vi "Build Array String.vi"() -> ()   [LabVIEW 2010]
panel:
  out "new string":string="CP_Data[000]=0x00\\r\nCP_Data[001]=0x00\\r\nCP_Data[002]=0x00\\r\nCP_Data[003]=0x00\\r\nCP_Data[004]=0x00\\r\nCP_Data[005]=0x00\\r\nCP_Data[006]=0x00\\r\nCP_Data[007]=0x00\\r\nCP_Data[008]=0x00\\r\nCP_Data[009]=0x00\\r\nCP_Data[010]=0x00\\r\nCP_Data[011]=0x00\\r\nCP_Data[012]=0x00\\r\nCP_Data[013]=0x00\\r\nCP_Data[014]=0x00\\r\nCP_Data[015]=0x00\\r\nCP_Data[016]=0x00\\r\nCP_Data[017]=0x00\\r\nCP_Data[018]=0x00\\r\nCP_Data[019]=0x00\\r\nCP_Data[020]=0x00\\r\nCP_Data[021]=0x00\\r\nCP_Data[022]=0x00\\r\nCP_Data[023]=0x00\\r\nCP_Data[024]=0x00\\r\nCP_Data[025]=0x00\\r\nCP_Data[026]=0x00\\r\nCP_Data[027]=0x00\\r\nCP_Data[028]=0x00\\r\nCP_Data[029]=0x00\\r\nCP_Data[030]=0x00\\r\nCP_Data[031]=0x00\\r\nCP_Data[032]=0x00\\r\nCP_Data[033]=0x00\\r\nCP_Data[034]=0x00\\r\nCP_Data[035]=0x00\\r\nCP_Data[036]=0x00\\r\nCP_Data[037]=0x00\\r\nCP_Data[038]=0x00\\r\nCP_Data[039]=0x00\\r\nCP_Data[040]=0x00\\r\nCP_Data[041]=0x00\\r\nCP_Data[042]=0x00\\r\nCP_Data[043]=0x00\\r\nCP_Data[044]=0x00\\r\nCP_Data[045]=0x00\\r\nCP_Data[046]=0x00\\r\nCP_Data[047]=0x00\\r\nCP_Data[048]=0x00\\r\nCP_Data[049]=0x00\\r\nCP_Data[050]=0x00\\r\nCP_Data[051]=0x00\\r\nCP_Data[052]=0x00\\r\nCP_Data[053]=0x00\\r\nCP_Data[054]=0x00\\r\nCP_Data[055]=0x00\\r\nCP_Data[056]=0x00\\r\nCP_Data[057]=0x00\\r\nCP_Data[058]=0x00\\r\nCP_Data[059]=0x00\\r\nCP_Data[060]=0x00\\r\nCP_Data[061]=0x00\\r\nCP_Data[062]=0x00\\r\nCP_Data[063]=0x00\\r\nCP_Data[064]=0x00\\r\nCP_Data[065]=0x00\\r\nCP_Data[066]=0x00\\r\nCP_Data[067]=0x00\\r\nCP_Data[068]=0x00\\r\nCP_Data[069]=0x00\\r\nCP_Data[070]=0x00\\r\nCP_Data[071]=0x00\\r\nCP_Data[072]=0x00\\r\nCP_Data[073]=0x00\\r\nCP_Data[074]=0x00\\r\nCP_Data[075]=0x00\\r\nCP_Data[076]=0x00\\r\nCP_Data[077]=0x00\\r\nCP_Data[078]=0x00\\r\nCP_Data[079]=0x00\\r\nCP_Data[080]=0x00\\r\nCP_Data[081]=0x00\\r\nCP_Data[082]=0x00\\r\nCP_Data[083]=0x00\\r\nCP_Data[084]=0x00\\r\nCP_Data[085]=0x00\\r\nCP_Data[086]=0x00\\r\nCP_Data[087]=0x00\\r\nCP_Data[088]=0x00\\r\nCP_Data[089]=0x00\\r\nCP_Data[090]=0x00\\r\nCP_Data[091]=0x00\\r\nCP_Data[092]=0x00\\r\nCP_Data[093]=0x00\\r\nCP_Data[094]=0x00\\r\nCP_Data[095]=0x00\\r\nCP_Data[096]=0x00\\r\nCP_Data[097]=0x00\\r\nCP_Data[098]=0x00\\r\nCP_Data[099]=0x00\\r\nCP_Data[100]=0x00\\r\nCP_Data[101]=0x00\\r\nCP_Data[102]=0x00\\r\nCP_Data[103]=0x00\\r\nCP_Data[104]=0x00\\r\nCP_Data[105]=0x00\\r\nCP_Data[106]=0x00\\r\nCP_Data[107]=0x00\\r\nCP_Data[108]=0x00\\r\nCP_Data[109]=0x00\\r\nCP_Data[110]=0x00\\r\nCP_Data[111]=0x00\\r\nCP_Data[112]=0x00\\r\nCP_Data[113]=0x00\\r\nCP_Data[114]=0x00\\r\nCP_Data[115]=0x00\\r\nCP_Data[116]=0x00\\r\nCP_Data[117]=0x00\\r\nCP_Data[118]=0x00\\r\nCP_Data[119]=0x00\\r\nCP_Data[120]=0x00\\r\nCP_Data[121]=0x00\\r\nCP_Data[122]=0x00\\r\nCP_Data[123]=0x00\\r\nCP_Data[124]=0x00\\r\nCP_Data[125]=0x00\\r\nCP_Data[126]=0x00\\r\nCP_Data[127]=0x00\\r\nCP_Data[128]=0x00\\r\nCP_Data[129]=0x00\\r\nCP_Data[130]=0x00\\r\nCP_Data[131]=0x00\\r\nCP_Data[132]=0x00\\r\nCP_Data[133]=0x00\\r\nCP_Data[134]=0x00\\r\nCP_Data[135]=0x00\\r\nCP_Data[136]=0x00\\r\nCP_Data[137]=0x00\\r\nCP_Data[138]=0x00\\r\nCP_Data[139]=0x00\\r\nCP_Data[140]=0x00\\r\nCP_Data[141]=0x00\\r\nCP_Data[142]=0x00\\r\nCP_Data[143]=0x00\\r\nCP_Data[144]=0x00\\r\nCP_Data[145]=0x00\\r\nCP_Data[146]=0x00\\r\nCP_Data[147]=0x00\\r\nCP_Data[148]=0x00\\r\nCP_Data[149]=0x00\\r\nCP_Data[150]=0x00\\r\nCP_Data[151]=0x00\\r\nCP_Data[152]=0x00\\r\nCP_Data[153]=0x00\\r\nCP_Data[154]=0x00\\r\nCP_Data[155]=0x00\\r\nCP_Data[156]=0x00\\r\nCP_Data[157]=0x00\\r\nCP_Data[158]=0x00\\r\nCP_Data[159]=0x00\\r\nCP_Data[160]=0x00\\r\nCP_Data[161]=0x00\\r\nCP_Data[162]=0x00\\r\nCP_Data[163]=0x00\\r\nCP_Data[164]=0x00\\r\nCP_Data[165]=0x00\\r\nCP_Data[166]=0x00\\r\nCP_Data[167]=0x00\\r\nCP_Data[168]=0x00\\r\nCP_Data[169]=0x00\\r\nCP_Data[170]=0x00\\r\nCP_Data[171]=0x00\\r\nCP_Data[172]=0x00\\r\nCP_Data[173]=0x00\\r\nCP_Data[174]=0x00\\r\nCP_Data[175]=0x00\\r\nCP_Data[176]=0x00\\r\nCP_Data[177]=0x00\\r\nCP_Data[178]=0x00\\r\nCP_Data[179]=0x00\\r\nCP_Data[180]=0x00\\r\nCP_Data[181]=0x00\\r\nCP_Data[182]=0x00\\r\nCP_Data[183]=0x00\\r\nCP_Data[184]=0x00\\r\nCP_Data[185]=0x00\\r\nCP_Data[186]=0x00\\r\nCP_Data[187]=0x00\\r\nCP_Data[188]=0x00\\r\nCP_Data[189]=0x00\\r\nCP_Data[190]=0x00\\r\nCP_Data[191]=0x00\\r\nCP_Data[192]=0x00\\r\nCP_Data[193]=0x00\\r\nCP_Data[194]=0x00\\r\nCP_Data[195]=0x00\\r\nCP_Data[196]=0x00\\r\nCP_Data[197]=0x00\\r\nCP_Data[198]=0x00\\r\nCP_Data[199]=0x00\\r\nCP_Data[200]=0x00\\r\nCP_Data[201]=0x00\\r\nCP_Data[202]=0x00\\r\nCP_Data[203]=0x00\\r\nCP_Data[204]=0x00\\r\nCP_Data[205]=0x00\\r\nCP_Data[206]=0x00\\r\nCP_Data[207]=0x00\\r\nCP_Data[208]=0x00\\r\nCP_Data[209]=0x00\\r\nCP_Data[210]=0x00\\r\nCP_Data[211]=0x00\\r\nCP_Data[212]=0x00\\r\nCP_Data[213]=0x00\\r\nCP_Data[214]=0x00\\r\nCP_Data[215]=0x00\\r\nCP_Data[216]=0x00\\r\nCP_Data[217]=0x00\\r\nCP_Data[218]=0x00\\r\nCP_Data[219]=0x00\\r\nCP_Data[220]=0x00\\r\nCP_Data[221]=0x00\\r\nCP_Data[222]=0x00\\r\nCP_Data[223]=0x00\\r\nCP_Data[224]=0x00\\r\nCP_Data[225]=0x00\\r\nCP_Data[226]=0x00\\r\nCP_Data[227]=0x00\\r\nCP_Data[228]=0x00\\r\nCP_Data[229]=0x00\\r\nCP_Data[230]=0x00\\r\nCP_Data[231]=0x00\\r\nCP_Data[232]=0x00\\r\nCP_Data[233]=0x00\\r\nCP_Data[234]=0x00\\r\nCP_Data[235]=0x00\\r\nCP_Data[236]=0x00\\r\nCP_Data[237]=0x00\\r\nCP_Data[238]=0x00\\r\nCP_Data[239]=0x00\\r\nCP_Data[240]=0x00\\r\nCP_Data[241]=0x00\\r\nCP_Data[242]=0x00\\r\nCP_Data[243]=0x00\\r\nCP_Data[244]=0x00\\r\nCP_Data[245]=0x00\\r\nCP_Data[246]=0x00\\r\nCP_Data[247]=0x00\\r\nCP_Data[248]=0x00\\r\nCP_Data[249]=0x00\\r\nCP_Data[250]=0x00\\r\nCP_Data[251]=0x00\\r\nCP_Data[252]=0x00\\r\nCP_Data[253]=0x00\\r\nCP_Data[254]=0x00\\r\n"
  in  "head":string
  in  "N":i32=255
  in  "format string":string="%03d]=0x00\\\\r\n"
  in  "prefix":string="CP_Data["
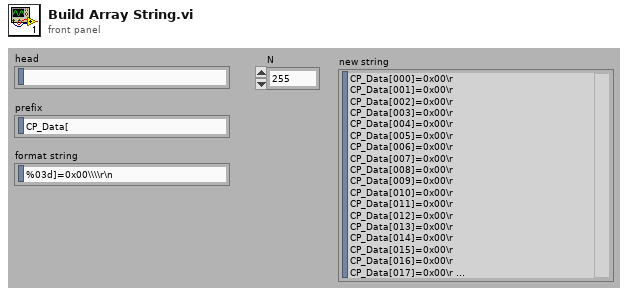
[diagram p1: front panel]
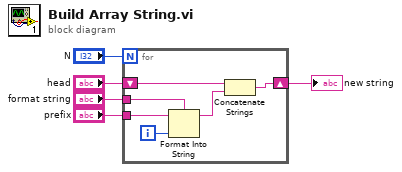
[diagram p0: block diagram]
diagram:
  n1 = for {
    N: "N" -> [_]
    tunnel: "prefix" -> [w11]
    tunnel: "format string" -> [w10]
    shift-right: [w6] -> w1
    shift-left: "head" -> [w7]
    i -> [w9]
    n2 = Format Into String(format string=w10, initial string=w11, w9) -> (resulting string=w8:string)  [unwired: 1 in, 1 out]
    n3 = Concatenate Strings(w7, w8) -> (w6:string)
  }
  "new string" <- w1
